vi "设置模块队列名.vi"() -> (2 "Msg":string)   [LabVIEW 2016, in "斯坦道氨氮.lvlib"]
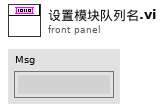
[diagram p1: front panel]
types:
  T1 = cluster{"COD":bool, "氨氮":bool, "总氮":bool, "总磷":bool}
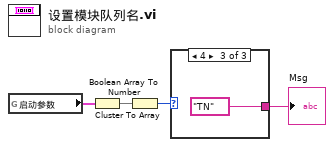
[diagram p0: block diagram]
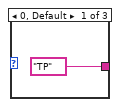
[diagram p2: hidden frame]
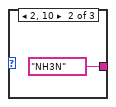
[diagram p3: hidden frame]
diagram:
  n1 = global read "总磷总氮断电保存全局变量.vi" "启动参数"() -> (w4:T1)
  n2 = Cluster To Array(cluster=w4) -> (array=w3:bool[])
  n3 = Boolean Array To Number(Boolean array=w3) -> (number=w2:u32)
  n4 = case shown="4" w2 {
    tunnel: ["TP" ("队列名") "NH3N" ("队列名") "TN" ("队列名")] -> w1
    frame 0, Default {
    }
    frame 2, 10 {
    }
    frame 4 {
    }
  }
  "Msg" <- w1
